vi "Array-Evaluate MATLAB Expression.vi"(0 "Expression":string, 7 "UserVars":T1[](array[typedef]), 11 "error in":errorcluster) -> (4 "Result (1D)":dbl[](array[numeric]), 15 "error out":errorcluster)   [LabVIEW 2015]
uses:
  Tosca/LV Source/Typedefs/Tosca-Rove Variable.ctl
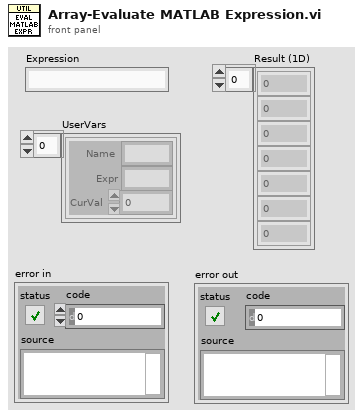
[diagram p1: front panel]
types:
  T1 = typedef "Tosca-Rove Variable.ctl" = cluster{"Name":string, "Expr":string, "CurVal":dbl}
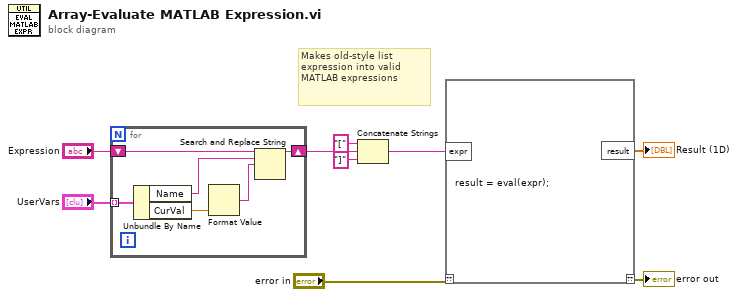
[diagram p0: block diagram]
diagram:
  # "Makes old-style list expression into valid MATLAB expressions"
  n1 = for {
    tunnel: "UserVars" -> [w15] mode=indexing
    shift-right: [w10] -> w7
    shift-left: "Expression" -> [w14]
    n2 = Unbundle By Name(w15) -> ("Name"=w13:string, "CurVal"=w12:dbl)
    n3 = Format Value(value (0)=w12) -> (output string=w11:string)  [unwired: 2 in]
    n4 = Search and Replace String(input string=w14, search string=w13, replace string=w11) -> (result string=w10:string)  [unwired: 5 in, 3 out]
  }
  n5 = Concatenate Strings("[" ("string"), w7, "]" ("string")) -> (w4:string)
  n6 = script code="result = eval(expr);"("??"="error in", "expr"=w4) -> ("??"=→"error out":errorcluster, "result"=→"Result (1D)":dbl[])
